vi "Set Exclusions By Path.vi"(8 "error in (no error)":errorcluster, 10 "Path exclusions":T1={"Exclude files from vi.lib"=TRUE, "Exclude files from instr.lib"=TRUE, "Exclude files from user.lib"=TRUE}, 11 "SDIST in":refnum<class "NI_AB_API_SDIST.lvclass">) -> (0 "error out":errorcluster, 3 "SDIST out":refnum<class "NI_AB_API_SDIST.lvclass">)   [LabVIEW 2020, in "NI_AB_API_SDIST.lvclass"]
uses:
  <vilib>/AppBuilder/AB_API/SDIST/NI_AB_API_SDIST.lvclass
  <vilib>/AppBuilder/AB_API/common/AB_API Path Exclusions.ctl
  <vilib>/AppBuilder/AB_API/Build/NI_AB_API_Build.lvclass
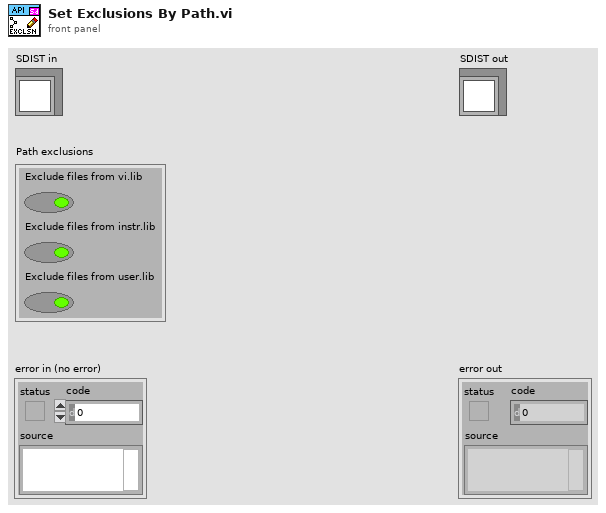
[diagram p1: front panel]
types:
  T1 = typedef "AB_API Path Exclusions.ctl" = cluster{"Exclude files from vi.lib":bool, "Exclude files from instr.lib":bool, "Exclude files from user.lib":bool}
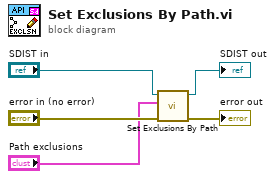
[diagram p0: block diagram]
diagram:
  n1 = call-parent "Set Exclusions By Path.vi"("error in (no error)"="error in (no error)", "Path exclusions"="Path exclusions", "NI_AB_API_Build in"="SDIST in") -> ("error out"=→"error out":errorcluster, "NI_AB_API_Build out"=→"SDIST out":refnum<class "NI_AB_API_SDIST.lvclass">)  [unwired: 7 in]
